vi "RTS Set Test End Time.vi"(0 "Current Test":T1={"Chamber 1-3"=[{"End Time"=timestamp(3594046716.8947463 s since 1904-01-01), "Start Time"=timestamp(3593614713.19836 s since 1904-01-01), "Door Opening Schedule:"={"Open Door Timer (s)"=12.0, "Delay Time (s)"=695.0, "Close Door Timer (s)"=12.0}, "Enable Door Ops"=TRUE, "Door Openings"=120, "Temp (°F)"=0.0, "Humidity (%)"=0.0, "Voltage (V)"=0.0, "Door Open Sequence:"=enum."", "Door Delay(sec)"=0.0, "Dehum (°F)"=0.0, "Cool (°F)"=0.0}], "Chamber 1-2"=[{"End Time"=timestamp(3594046708.565822 s since 1904-01-01), "Start Time"=timestamp(3593614700.612354 s since 1904-01-01), "Door Opening Schedule:"={"Open Door Timer (s)"=12.0, "Delay Time (s)"=695.0, "Close Door Timer (s)"=12.0}, "Enable Door Ops"=TRUE, "Door Openings"=0, "Temp (°F)"=0.0, "Humidity (%)"=0.0, "Voltage (V)"=0.0, "Door Open Sequence:"=enum."", "Door Delay(sec)"=0.0, "Dehum (°F)"=0.0, "Cool (°F)"=0.0}], "Chamber 1-1"=[{"End Time"=timestamp(3594046691.867131 s since 1904-01-01), "Start Time"=timestamp(3593614687.850203 s since 1904-01-01), "Door Opening Schedule:"={"Open Door Timer (s)"=12.0, "Delay Time (s)"=2800.0, "Close Door Timer (s)"=12.0}, "Enable Door Ops"=TRUE, "Door Openings"=30, "Temp (°F)"=0.0, "Humidity (%)"=0.0, "Voltage (V)"=0.0, "Door Open Sequence:"=enum."", "Door Delay(sec)"=0.0, "Dehum (°F)"=0.0, "Cool (°F)"=0.0}], "Standard Tests 1-1"=enum."511-B111 Internal Moisture"} {"Chamber 1-1"."Start Time" format="%<%X\n%x>T"; "Chamber 1-1"."End Time" format="%<%X\n%x>T"; "Chamber 1-2"."Start Time" format="%<%X\n%x>T"; "Chamber 1-2"."End Time" format="%<%X\n%x>T"; "Chamber 1-3"."Start Time" format="%<%X\n%x>T"; "Chamber 1-3"."End Time" format="%<%X\n%x>T"}, 2 "Operation Duration (hrs)":dbl=57600.0 format="%#_13g", 11 "Error In":errorcluster, 12 "index":i32) -> (4 "Current Test Output":T1={"Chamber 1-3"=[{"End Time"=timestamp(3594046716.8947463 s since 1904-01-01), "Start Time"=timestamp(3593614713.19836 s since 1904-01-01), "Door Opening Schedule:"={"Open Door Timer (s)"=12.0, "Delay Time (s)"=695.0, "Close Door Timer (s)"=12.0}, "Enable Door Ops"=TRUE, "Door Openings"=120, "Temp (°F)"=0.0, "Humidity (%)"=0.0, "Voltage (V)"=0.0, "Door Open Sequence:"=enum."", "Door Delay(sec)"=0.0, "Dehum (°F)"=0.0, "Cool (°F)"=0.0}], "Chamber 1-2"=[{"End Time"=timestamp(3594046708.565822 s since 1904-01-01), "Start Time"=timestamp(3593614700.612354 s since 1904-01-01), "Door Opening Schedule:"={"Open Door Timer (s)"=12.0, "Delay Time (s)"=695.0, "Close Door Timer (s)"=12.0}, "Enable Door Ops"=TRUE, "Door Openings"=0, "Temp (°F)"=0.0, "Humidity (%)"=0.0, "Voltage (V)"=0.0, "Door Open Sequence:"=enum."", "Door Delay(sec)"=0.0, "Dehum (°F)"=0.0, "Cool (°F)"=0.0}], "Chamber 1-1"=[{"End Time"=timestamp(3594046691.867131 s since 1904-01-01), "Start Time"=timestamp(3593614687.850203 s since 1904-01-01), "Door Opening Schedule:"={"Open Door Timer (s)"=12.0, "Delay Time (s)"=2800.0, "Close Door Timer (s)"=12.0}, "Enable Door Ops"=TRUE, "Door Openings"=30, "Temp (°F)"=0.0, "Humidity (%)"=0.0, "Voltage (V)"=0.0, "Door Open Sequence:"=enum."", "Door Delay(sec)"=0.0, "Dehum (°F)"=0.0, "Cool (°F)"=0.0}], "Standard Tests 1-1"=enum."511-B111 Internal Moisture"} {"Chamber 1-1"."Start Time" format="%<%X\n%x>T"; "Chamber 1-1"."End Time" format="%<%X\n%x>T"; "Chamber 1-2"."Start Time" format="%<%X\n%x>T"; "Chamber 1-2"."End Time" format="%<%X\n%x>T"; "Chamber 1-3"."Start Time" format="%<%X\n%x>T"; "Chamber 1-3"."End Time" format="%<%X\n%x>T"}, 15 "Error Out":errorcluster)   [LabVIEW 2016]
uses:
  Type Definitions/RTS Door Op Data.ctl
  Type Definitions/RTS Door Ops Client.ctl
  Type Definitions/RTS Door Opening Schedule.ctl
  Type Definitions/RTS Door Ops Sequence.ctl
  Type Definitions/RTS Standard Door Opening Test.ctl
panel:
  # "Chamber Conditions:"
  # "Chamber Conditions:"
  # "Chamber Conditions:"
  # "Chamber Conditions:"
  # "Chamber Conditions:"
  # "Chamber Conditions:"
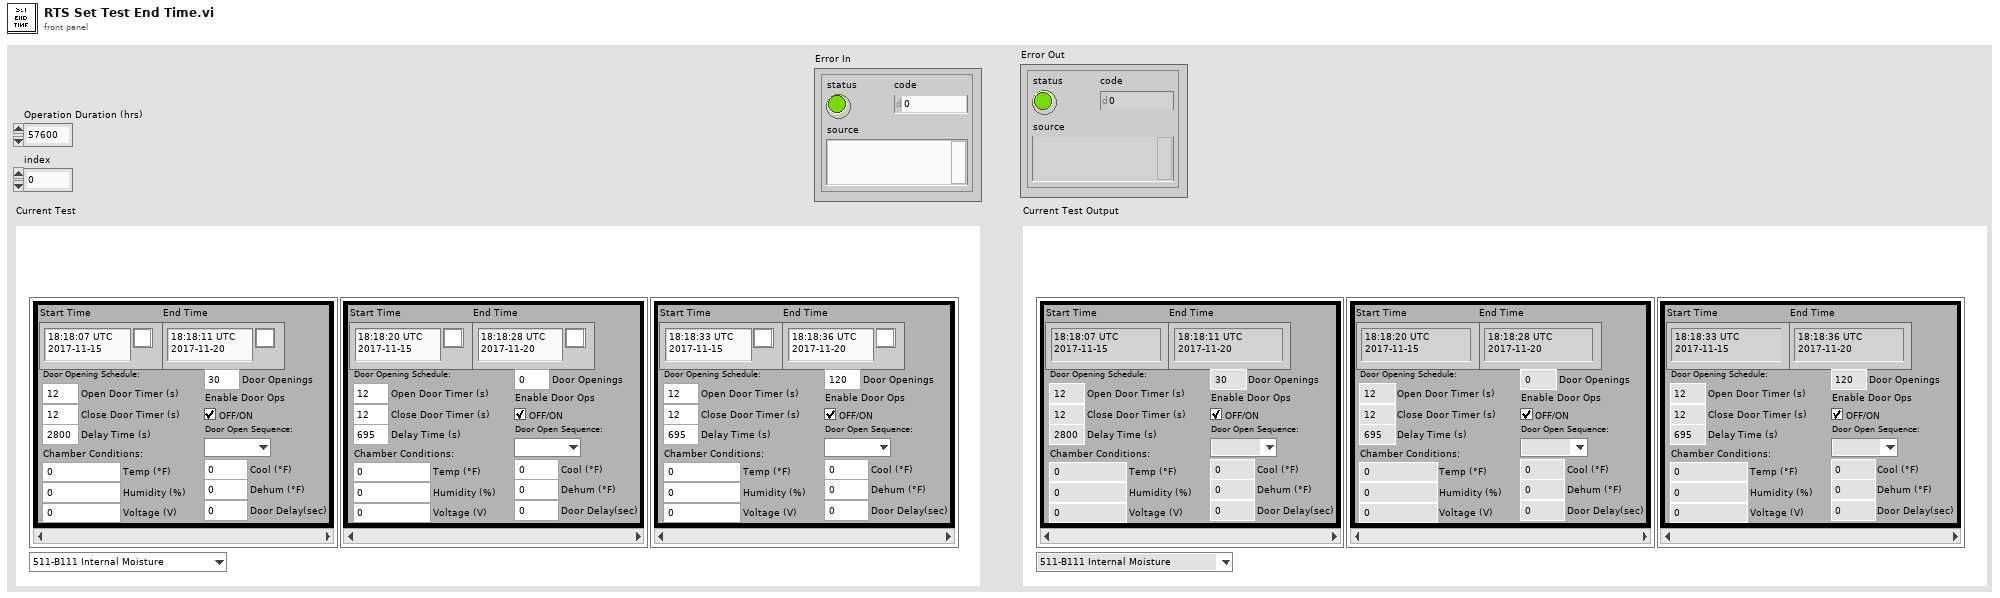
[diagram p1: front panel]
types:
  T1 = typedef "RTS Door Op Data.ctl" = cluster{"Chamber 1-3":T2[], "Chamber 1-2":T2[], "Chamber 1-1":T2[], "Standard Tests 1-1":T5}
  T2 = typedef "RTS Door Ops Client.ctl" = cluster{"End Time":timestamp, "Start Time":timestamp, "Door Opening Schedule:":T3, "Enable Door Ops":bool, "Door Openings":u32, "Temp (°F)":dbl, "Humidity (%)":dbl, "Voltage (V)":dbl, "Door Open Sequence:":T4, "Door Delay(sec)":dbl, "Dehum (°F)":dbl, "Cool (°F)":dbl}
  T3 = typedef "RTS Door Opening Schedule.ctl" = cluster{"Open Door Timer (s)":dbl, "Delay Time (s)":dbl, "Close Door Timer (s)":dbl}
  T4 = typedef "RTS Door Ops Sequence.ctl" = enum16{"", "1st", "2nd", "3rd"}
  T5 = typedef "RTS Standard Door Opening Test.ctl" = enum16{"Standard ETPs", "511-B113 EHUT", "511-B110 HUT", "512-C410 SLAT", "511-B111 Internal Moisture", "511-C401 Moisture Accumulation", "511-B100 No Door Opening (NDO)", "511-B304 ISO Energy Consumption", "Custom Test", "Cancel Test"}
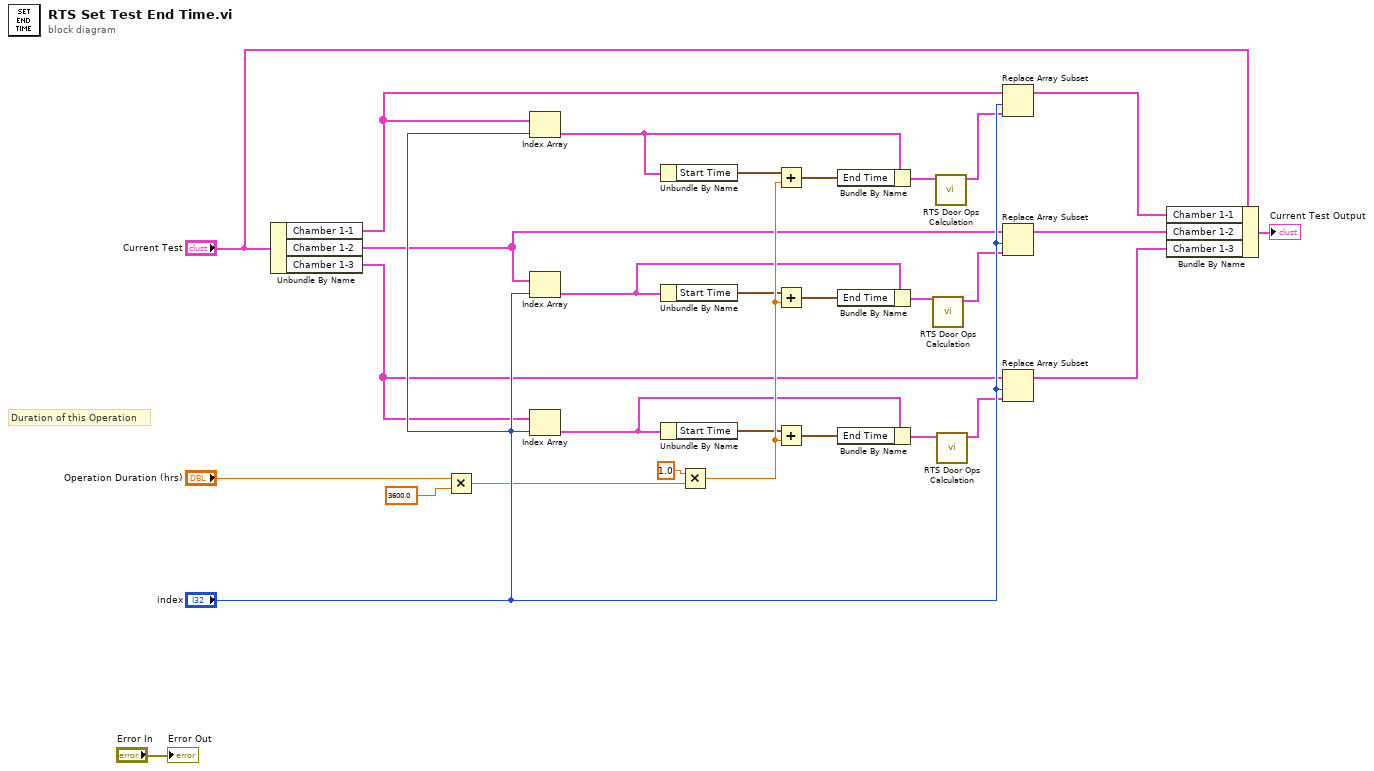
[diagram p0: block diagram]
diagram:
  # "Duration of this Operation"
  n1 = Unbundle By Name("Current Test") -> ("Chamber 1-1"=w10:T2[], "Chamber 1-2"=w12:T2[], "Chamber 1-3"=w11:T2[])
  n2 = Multiply(x="Operation Duration (hrs)", y=3600.0) -> (x*y=w1:dbl)
  n3 = Index Array(array=w10, index="index") -> (element=w21:T2)
  n4 = Index Array(array=w12, index="index") -> (element=w19:T2)
  n5 = Index Array(array=w11, index="index") -> (element=w18:T2)
  n6 = Unbundle By Name(w21) -> ("Start Time"=w25:timestamp)
  n7 = Unbundle By Name(w19) -> ("Start Time"=w24:timestamp)
  n8 = Unbundle By Name(w18) -> ("Start Time"=w23:timestamp)
  n9 = Multiply(x=1.0, y=w1) -> (x*y=w30:dbl)
  n10 = Add(x=w25, y=w30) -> (x+y=w26:timestamp)
  n11 = Add(x=w24, y=w30) -> (x+y=w27:timestamp)
  n12 = Add(x=w23, y=w30) -> (x+y=w28:timestamp)
  n13 = Bundle By Name(cluster=w21, "End Time"=w26) -> (w5:T2)
  n14 = Bundle By Name(cluster=w19, "End Time"=w27) -> (w7:T2)
  n15 = Bundle By Name(cluster=w18, "End Time"=w28) -> (w9:T2)
  n16 = call "RTS Door Ops Calculation.vi"("Chamber 1-1 in"=w7) -> ("Chamber 1-1 out"=w6:T2)  [unwired: 9 in, 1 out]
  n17 = call "RTS Door Ops Calculation.vi"("Chamber 1-1 in"=w5) -> ("Chamber 1-1 out"=w4:T2)  [unwired: 9 in, 1 out]
  n18 = call "RTS Door Ops Calculation.vi"("Chamber 1-1 in"=w9) -> ("Chamber 1-1 out"=w8:T2)  [unwired: 9 in, 1 out]
  n19 = Replace Array Subset(array=w10, new element=w4, index="index") -> (w16:T2[])
  n20 = Replace Array Subset(array=w12, new element=w6, index="index") -> (w15:T2[])
  n21 = Replace Array Subset(array=w11, new element=w8, index="index") -> (w14:T2[])
  n22 = Bundle By Name(cluster="Current Test", "Chamber 1-1"=w16, "Chamber 1-2"=w15, "Chamber 1-3"=w14) -> (→"Current Test Output":T1)
  "Error Out" <- "Error In"
